vi "Redraw__LCR.vi"(8 "error in (no error)":errorcluster, 10 "BX.FP Refs":T9, 11 "State":T1={"Orientation"=0, "ActivePicture"={"image type"=0, "image depth"=0, "image"=[], "mask"=[], "colors"=[], "Rectangle"={"left"=0, "top"=0, "right"=0, "bottom"=0}}, "Pictures"={"Normal"={"image type"=0, "image depth"=0, "image"=[], "mask"=[], "colors"=[], "Rectangle"={"left"=0, "top"=0, "right"=0, "bottom"=0}}, "Hilite"={"image type"=0, "image depth"=0, "image"=[], "mask"=[], "colors"=[], "Rectangle"={"left"=0, "top"=0, "right"=0, "bottom"=0}}}, "Text"={"String"="", "Font"={"Font Name:"="", "Size"=0, "Strikeout?"=FALSE, "Italic?"=FALSE, "Underline?"=FALSE, "Outline?"=FALSE, "Shadow?"=FALSE, "Bold?"=FALSE}, "TextColor"=0}, "RunTimeSettings"={"Highlight"=FALSE, "ShowButton"=TRUE, "Behaviour"=enum."Switch when pressed", "React if disabled"=FALSE, "Nudge Button"=TRUE, "ShowButton on Hover"=FALSE, "Button Type"=enum."System"}, "Messages"=[], "Status"=0, "XControl Label"="", "Boolean Value"=FALSE} {"Status" format="%.0x"}) -> (0 "error out":errorcluster, 3 "State Out":T1={"Orientation"=0, "ActivePicture"={"image type"=0, "image depth"=0, "image"=[], "mask"=[], "colors"=[], "Rectangle"={"left"=0, "top"=0, "right"=0, "bottom"=0}}, "Pictures"={"Normal"={"image type"=0, "image depth"=0, "image"=[], "mask"=[], "colors"=[], "Rectangle"={"left"=0, "top"=0, "right"=0, "bottom"=0}}, "Hilite"={"image type"=0, "image depth"=0, "image"=[], "mask"=[], "colors"=[], "Rectangle"={"left"=0, "top"=0, "right"=0, "bottom"=0}}}, "Text"={"String"="", "Font"={"Font Name:"="", "Size"=0, "Strikeout?"=FALSE, "Italic?"=FALSE, "Underline?"=FALSE, "Outline?"=FALSE, "Shadow?"=FALSE, "Bold?"=FALSE}, "TextColor"=0}, "RunTimeSettings"={"Highlight"=FALSE, "ShowButton"=TRUE, "Behaviour"=enum."Switch when pressed", "React if disabled"=FALSE, "Nudge Button"=TRUE, "ShowButton on Hover"=FALSE, "Button Type"=enum."System"}, "Messages"=[], "Status"=0, "XControl Label"="", "Boolean Value"=FALSE} caption="State" {"Status" format="%.0x"})   [LabVIEW 2011, in "BooleanXControl__LCR.xctl"]
doc: "This VI redraws the BX"
uses:
  BooleanXControl__LCR.xctl
  Abilities/BX.State__LCR.ctl
  Controls/BX.Orientation__LCR.ctl
  <vilib>/picture/picture.llb/imagedata.ctl
  Controls/BX.RTSettings__LCR.ctl
  Controls/BX.Behaviour__LCR.ctl
  Controls/BX.ButtonType__LCR.ctl
  Controls/BX.Message__LCR.ctl
  Controls/BX.Commands__LCR.ctl
  Controls/BX.Refs__LCR.ctl
  <vilib>/Utility/miscctls.llb/LVBoundsTypeDef.ctl
  <vilib>/Utility/miscctls.llb/LVPositionTypeDef.ctl
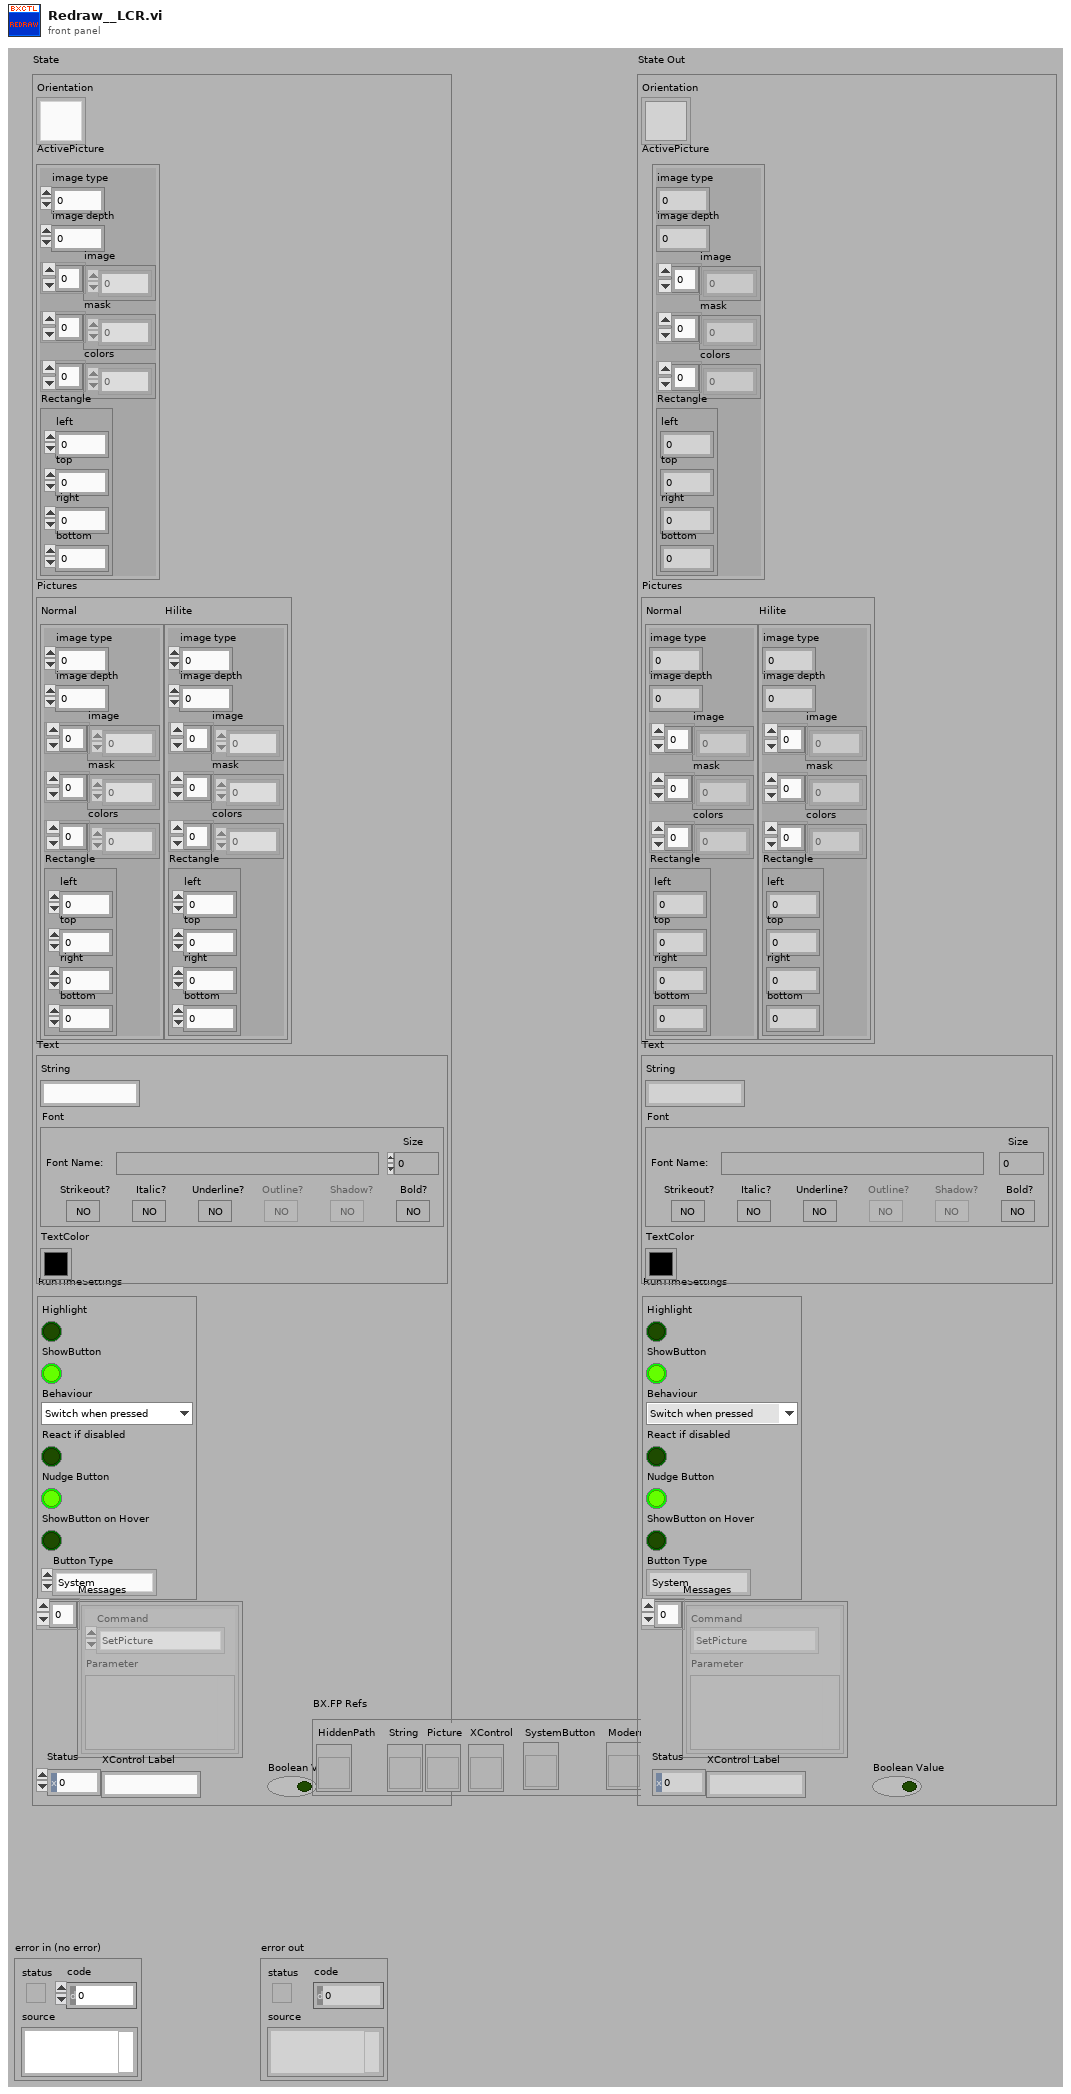
[diagram p1: front panel]
types:
  T1 = typedef "BooleanXControl__LCR.xctl/BX.State__LCR.ctl" = cluster{"Orientation":T2, "ActivePicture":T3, "Pictures":cluster{"Normal":T3, "Hilite":T3}, "Text":cluster{"String":string, "Font":cluster{"Font Name:":string, "Size":i16, "Strikeout?":bool, "Italic?":bool, "Underline?":bool, "Outline?":bool, "Shadow?":bool, "Bold?":bool}, "TextColor":u32}, "RunTimeSettings":T4, "Messages":T7[], "Status":u16, "XControl Label":string, "Boolean Value":bool}
  T2 = typedef "BooleanXControl__LCR.xctl/BX.Orientation__LCR.ctl" = u8
  T3 = typedef "imagedata.ctl" = cluster{"image type":i32, "image depth":i32, "image":u8[], "mask":u8[], "colors":u32[], "Rectangle":cluster{"left":i16, "top":i16, "right":i16, "bottom":i16}}
  T4 = typedef "BooleanXControl__LCR.xctl/BX.RTSettings__LCR.ctl" = cluster{"Highlight":bool, "ShowButton":bool, "Behaviour":T5, "React if disabled":bool, "Nudge Button":bool, "ShowButton on Hover":bool, "Button Type":T6}
  T5 = typedef "BooleanXControl__LCR.xctl/BX.Behaviour__LCR.ctl" = enum16{"Switch when pressed", "Switch when released", "Switch until released"}
  T6 = typedef "BooleanXControl__LCR.xctl/BX.ButtonType__LCR.ctl" = enum16{"System", "Modern", "Classic", "Decoration"}
  T7 = typedef "BooleanXControl__LCR.xctl/BX.Message__LCR.ctl" = cluster{"Command":T8, "Parameter":variant}
  T8 = typedef "BooleanXControl__LCR.xctl/BX.Commands__LCR.ctl" = enum16{"None", "SetPicture", "SetFont", "SetText", "SetOrientation", "Redraw", "SetTextColor", "SetRTSettings", "MultipleUpdate", "RT.Button", "RT.Hilite", "RT.Behaviour", "RT.Disabled", "ShowGUI", "RT.Nudge", "RT.Hover", "RT.ButtonType"}
  T9 = typedef "BooleanXControl__LCR.xctl/BX.Refs__LCR.ctl" = cluster{"HiddenPath":refnum<vi>, "String":refnum<vi>, "Picture":refnum<vi>, "XControl":refnum<vi>, "SystemButton":refnum<vi>, "ModernButton":refnum<vi>, "ClassicButton":refnum<vi>, "Decor Refnum":refnum<vi>}
  T10 = typedef "LVPositionTypeDef.ctl" = cluster{"Left":i32, "Top":i32}
  T11 = typedef "LVBoundsTypeDef.ctl" = cluster{"Width":u32, "Height":u32}
  T12 = cluster{"left":i16, "top":i16, "right":i16, "bottom":i16}
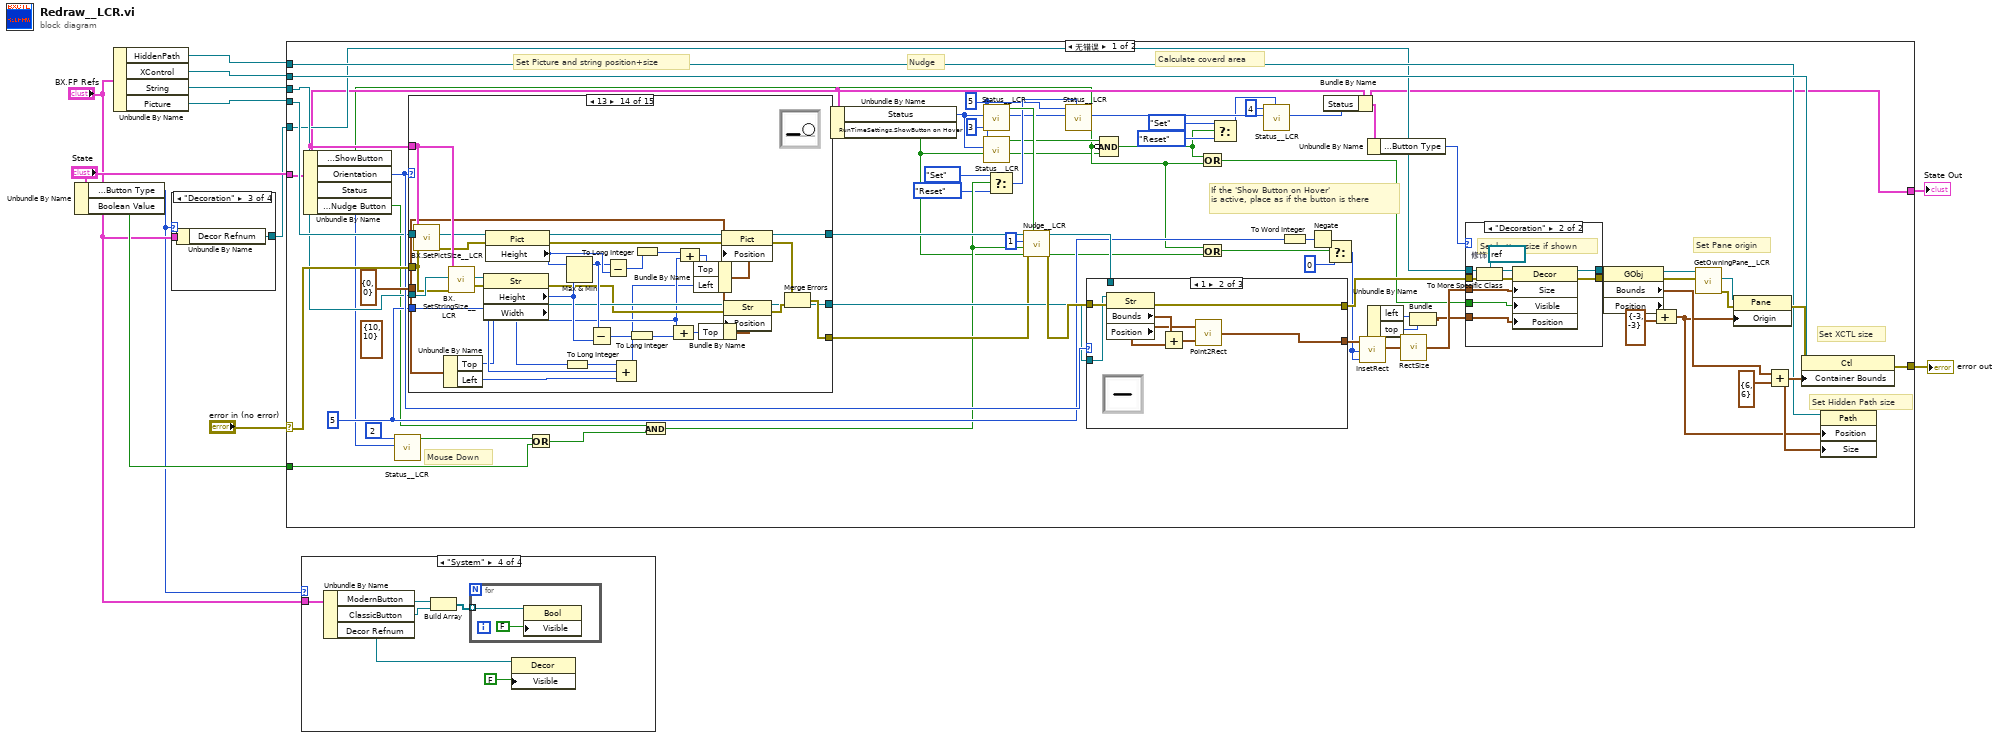
[diagram p0: block diagram]
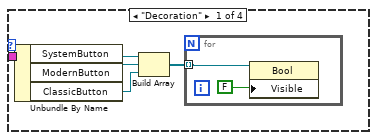
[diagram p2: hidden frame]
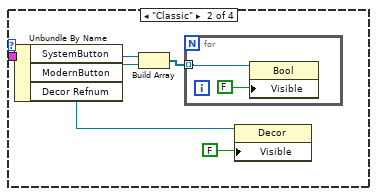
[diagram p3: hidden frame]
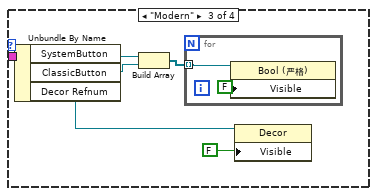
[diagram p4: hidden frame]
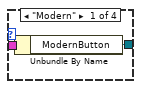
[diagram p5: hidden frame]
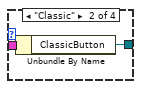
[diagram p6: hidden frame]
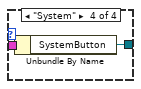
[diagram p7: hidden frame]
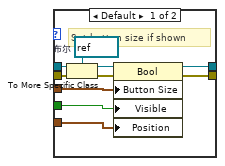
[diagram p8: hidden frame]
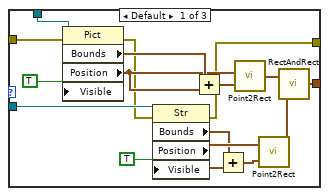
[diagram p9: hidden frame]
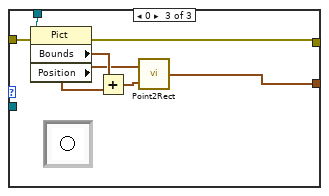
[diagram p10: hidden frame]
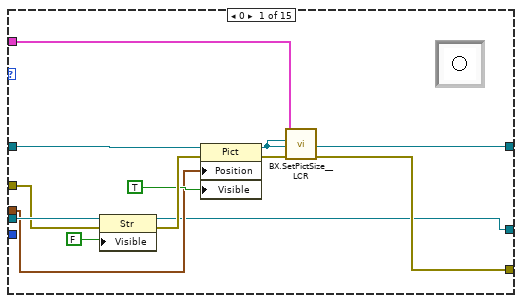
[diagram p11: hidden frame]
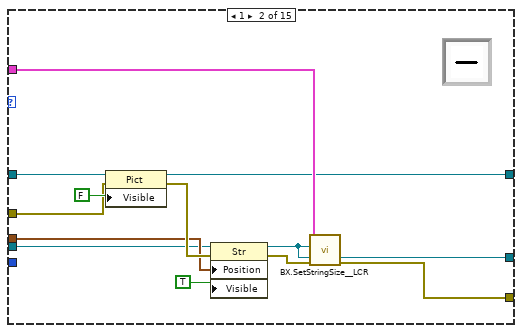
[diagram p12: hidden frame]
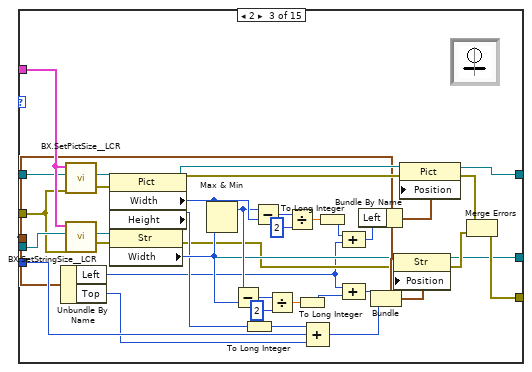
[diagram p13: hidden frame]
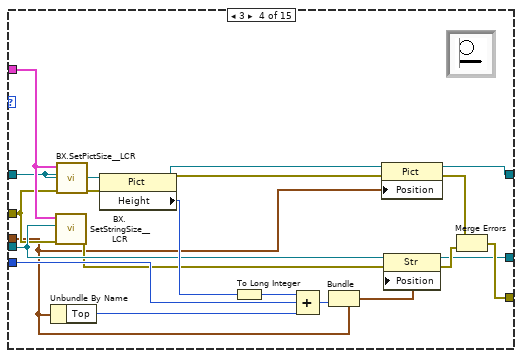
[diagram p14: hidden frame]
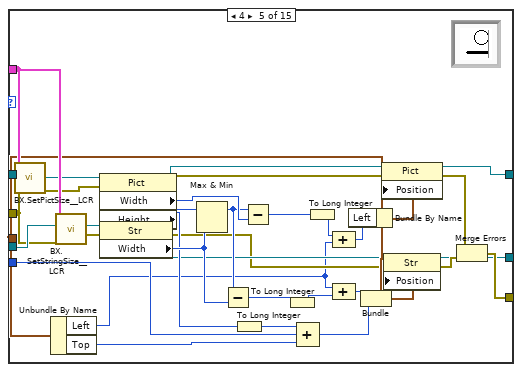
[diagram p15: hidden frame]
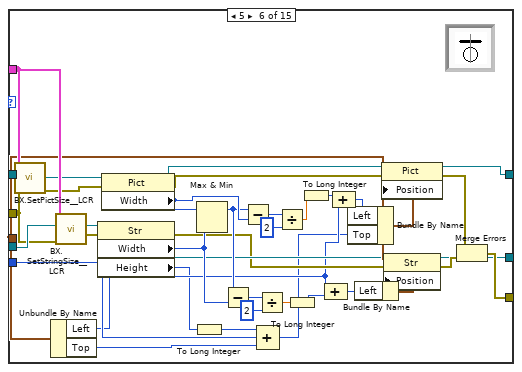
[diagram p16: hidden frame]
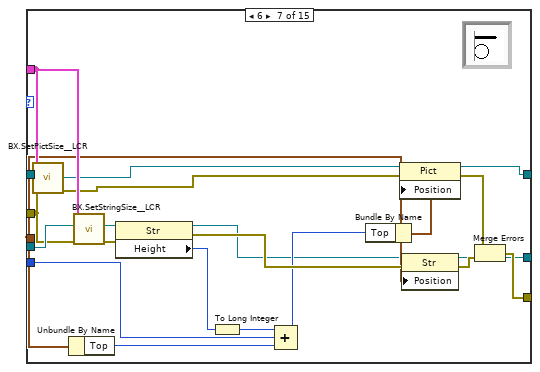
[diagram p17: hidden frame]
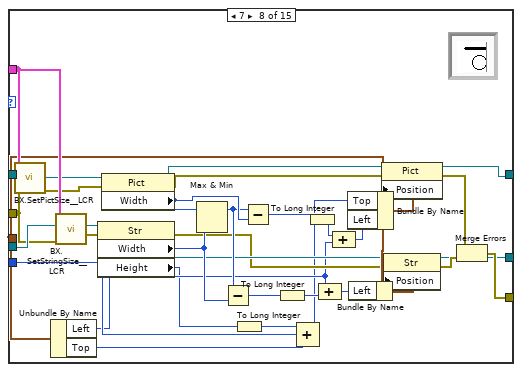
[diagram p18: hidden frame]
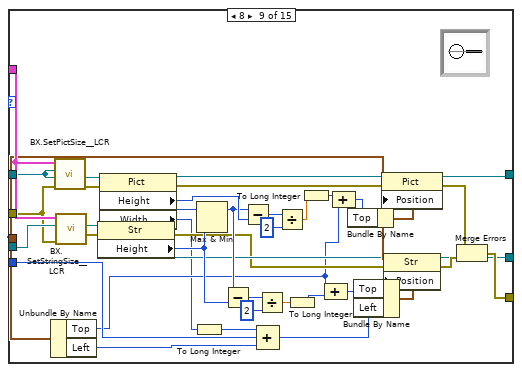
[diagram p19: hidden frame]
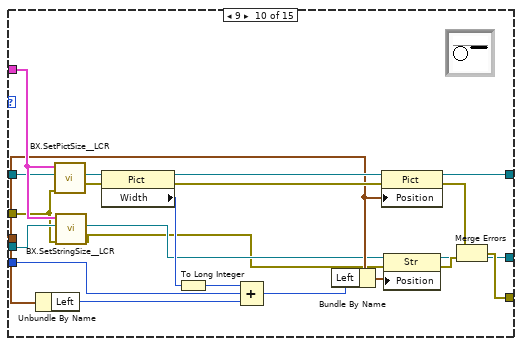
[diagram p20: hidden frame]
diagram:
  n1 = Unbundle By Name("State") -> ("RunTimeSettings.Button Type"=w1:T6, "Boolean Value"=w3:bool)
  n2 = Unbundle By Name("BX.FP Refs") -> ("HiddenPath"=w7:refnum<vi>, "XControl"=w8:refnum<vi>, "String"=w9:refnum<vi>, "Picture"=w10:refnum<vi>)
  n3 = case shown="\"Decoration\"" w1 {
    tunnel: "BX.FP Refs" -> [w14 w16 w18 w20]
    tunnel: [w13 w15 w17 w19] -> w4
    frame "Modern" {
      n4 = Unbundle By Name(w14) -> ("ModernButton"=w13:refnum<vi>)
    }
    frame "Classic" {
      n5 = Unbundle By Name(w16) -> ("ClassicButton"=w15:refnum<vi>)
    }
    frame "Decoration" {
      n6 = Unbundle By Name(w18) -> ("Decor Refnum"=w17:refnum<vi>)
    }
    frame "System" {
      n7 = Unbundle By Name(w20) -> ("SystemButton"=w19:refnum<vi>)
    }
  }
  n8 = case shown="无错误" "error in (no error)" {
    selector: "error in (no error)" -> [w74 w529]
    tunnel: [w77 w529] -> w11
    tunnel: "State" -> [w49 w528]
    tunnel: w10 -> [w62 _]
    tunnel: w4 -> [w51 _]
    tunnel: w9 -> [w61 _]
    tunnel: w8 -> [w66 _]
    tunnel: w7 -> [w65 _]
    tunnel: [w23 w528] -> w6
    tunnel: w3 -> [w21 _]
    frame No Error {
      (unwired) T10 {"Left"=10, "Top"=10} ("Position")
      w31 = u16 5 ("Bit")
      w56 = 5
      # "If the 'Show Button on Hover' \nis active, place as if the button is there"
      # "Mouse Down"
      # "Nudge"
      # "Set XCTL size"
      # "Set Hidden Path size"
      # "Set Pane origin"
      # "Calculate coverd area"
      # "Set Picture and string position+size"
      n9 = Unbundle By Name(w49) -> ("RunTimeSettings.ShowButton"=w27:bool, "Orientation"=w64:T2, "Status"=w53:u16, "RunTimeSettings.Nudge Button"=w52:bool)
      n10 = call "Status__LCR.vi"("Status In"=w53, "Bit"=u16 2 ("y")) -> ("Bit Value Out"=w24:bool)  [unwired: 8 in, 1 out]
      n11 = case shown="13" w64 {
        tunnel: w61 -> [w152 w155 w200 w208 w253 w290 w310 w343 w380 w386 w433 w470 w479 w523 w525]
        tunnel: w74 -> [w150 w163 w167 w205 w224 w257 w294 w314 w347 w384 w404 w437 w474 w494 w527]
        tunnel: T10 {"Left"=0, "Top"=0} ("Position") -> [w143 w161 w182 w204 w241 w273 w296 w332 w363 w387 w422 w453 w481 w512 _]
        tunnel: w62 -> [w148 w156 w198 w220 w251 w288 w299 w341 w378 w400 w431 w468 w480 w521 w526]
        tunnel: w49 -> [w146 w159 w201 w221 w254 w291 w311 w344 w381 w401 w434 w471 w491 w524 _]
        tunnel: [w144 w157 w175 w211 w234 w267 w304 w326 w357 w392 w416 w447 w487 w506 w527] -> w55
        tunnel: w56 -> [_ _ w184 w216 w243 w275 w308 w334 w365 w396 w424 w455 w490 w514 _]
        tunnel: [w142 w154 w166 w203 w223 w256 w293 w313 w346 w383 w403 w436 w473 w493 w526] -> w58
        tunnel: [w141 w153 w165 w202 w222 w255 w292 w312 w345 w382 w402 w435 w472 w492 w525] -> w60
        frame 0 {
          n12 = property class="Str"(reference=w152, error in=w150, "Visible"=FALSE) -> (reference out=w141:refnum<vi>, error out=w149:errorcluster)
          n13 = property class="Pict"(reference=w148, error in=w149, "Position"=w143, "Visible"=TRUE) -> (reference out=w142:refnum<vi>, error out=w145:errorcluster)
          n14 = call "BX.SetPictSize__LCR.vi"("error in (no error)"=w145, "Picture Control"=w142, "State"=w146) -> ("error out"=w144:errorcluster)  [unwired: 8 in]
        }
        frame 1 {
          n15 = property class="Pict"(reference=w156, error in=w163, "Visible"=FALSE) -> (reference out=w154:refnum<vi>, error out=w162:errorcluster)
          n16 = property class="Str"(reference=w155, error in=w162, "Position"=w161, "Visible"=TRUE) -> (reference out=w153:refnum<vi>, error out=w158:errorcluster)
          n17 = call "BX.SetStringSize__LCR.vi"("error in (no error)"=w158, "String Control"=w153, "State"=w159) -> ("error out"=w157:errorcluster)  [unwired: 8 in]
        }
        frame 2 {
          n18 = Unbundle By Name(w182) -> ("Left"=w168:i32, "Top"=w183:i32)
          n19 = call "BX.SetPictSize__LCR.vi"("error in (no error)"=w167, "Picture Control"=w198, "State"=w201) -> ("error out"=w197:errorcluster)  [unwired: 8 in]
          n20 = call "BX.SetStringSize__LCR.vi"("error in (no error)"=w167, "String Control"=w200, "State"=w201) -> ("error out"=w199:errorcluster)  [unwired: 8 in]
          n21 = property class="Pict"(reference=w198, error in=w197) -> (reference out=w187:refnum<vi>, error out=w186:errorcluster, "Width"=w196:u32, "Height"=w185:u32)
          n22 = property class="Str"(reference=w200, error in=w199) -> (reference out=w178:refnum<vi>, error out=w177:errorcluster, "Width"=w190:u32)
          n23 = Max & Min(x=w196, y=w190) -> (max(x,y)=w191:u32)  [unwired: 1 out]
          n24 = Subtract(x=w191, y=w190) -> (x-y=w192:u32)
          n25 = To Long Integer(number=w185) -> (32bit integer=w180:i32)
          n26 = Subtract(x=w191, y=w196) -> (x-y=w195:u32)
          n27 = Divide(x=w192, y=u32 2) -> (x/y=w188:dbl)
          n28 = Divide(x=w195, y=u32 2) -> (x/y=w189:dbl)
          n29 = To Long Integer(number=w188) -> (32bit integer=w170:i32)
          n30 = Compound Arithmetic op=ADD(w180, w184, w183) -> (w181:i32)
          n31 = To Long Integer(number=w189) -> (32bit integer=w172:i32)
          n32 = Compound Arithmetic op=ADD(w172, w168) -> (w171:i32)
          n33 = Compound Arithmetic op=ADD(w168, w170) -> (w169:i32)
          n34 = Bundle By Name(cluster=w182, "Left"=w171) -> (w179:T10)
          n35 = Bundle(cluster=w182, "Left"=w169, "Top"=w181) -> (w176:T10)
          n36 = property class="Str"(reference=w178, error in=w177, "Position"=w176) -> (reference out=w165:refnum<vi>, error out=w173:errorcluster)
          n37 = property class="Pict"(reference=w187, error in=w186, "Position"=w179) -> (reference out=w166:refnum<vi>, error out=w174:errorcluster)
          n38 = Merge Errors(w174, w173) -> (w175:errorcluster)
        }
        frame 3 {
          n39 = Unbundle By Name(w204) -> ("Top"=w215:i32)
          n40 = call "BX.SetStringSize__LCR.vi"("error in (no error)"=w205, "String Control"=w208, "State"=w221) -> ("error out"=w207:errorcluster)  [unwired: 8 in]
          n41 = call "BX.SetPictSize__LCR.vi"("error in (no error)"=w205, "Picture Control"=w220, "State"=w221) -> ("error out"=w206:errorcluster)  [unwired: 8 in]
          n42 = property class="Pict"(reference=w220, error in=w206) -> (reference out=w219:refnum<vi>, error out=w218:errorcluster, "Height"=w217:u32)
          n43 = To Long Integer(number=w217) -> (32bit integer=w213:i32)
          n44 = Compound Arithmetic op=ADD(w213, w216, w215) -> (w214:i32)
          n45 = Bundle(cluster=w204, "Top"=w214) -> (w212:T10)  [unwired: 1 in]
          n46 = property class="Pict"(reference=w219, error in=w218, "Position"=w204) -> (reference out=w203:refnum<vi>, error out=w210:errorcluster)
          n47 = property class="Str"(reference=w208, error in=w207, "Position"=w212) -> (reference out=w202:refnum<vi>, error out=w209:errorcluster)
          n48 = Merge Errors(w210, w209) -> (w211:errorcluster)
        }
        frame 4 {
          n49 = call "BX.SetPictSize__LCR.vi"("error in (no error)"=w224, "Picture Control"=w251, "State"=w254) -> ("error out"=w250:errorcluster)  [unwired: 8 in]
          n50 = Unbundle By Name(w241) -> ("Left"=w227:i32, "Top"=w242:i32)
          n51 = call "BX.SetStringSize__LCR.vi"("error in (no error)"=w224, "String Control"=w253, "State"=w254) -> ("error out"=w252:errorcluster)  [unwired: 8 in]
          n52 = property class="Pict"(reference=w251, error in=w250) -> (reference out=w246:refnum<vi>, error out=w245:errorcluster, "Width"=w249:u32, "Height"=w244:u32)
          n53 = property class="Str"(reference=w253, error in=w252) -> (reference out=w237:refnum<vi>, error out=w236:errorcluster, "Width"=w247:u32)
          n54 = Max & Min(x=w249, y=w247) -> (max(x,y)=w248:u32)  [unwired: 1 out]
          n55 = Subtract(x=w248, y=w247) -> (x-y=w225:u32)
          n56 = To Long Integer(number=w244) -> (32bit integer=w239:i32)
          n57 = Subtract(x=w248, y=w249) -> (x-y=w226:u32)
          n58 = To Long Integer(number=w225) -> (32bit integer=w229:i32)
          n59 = Compound Arithmetic op=ADD(w239, w243, w242) -> (w240:i32)
          n60 = To Long Integer(number=w226) -> (32bit integer=w231:i32)
          n61 = Compound Arithmetic op=ADD(w231, w227) -> (w230:i32)
          n62 = Compound Arithmetic op=ADD(w227, w229) -> (w228:i32)
          n63 = Bundle By Name(cluster=w241, "Left"=w230) -> (w238:T10)
          n64 = Bundle(cluster=w241, "Left"=w228, "Top"=w240) -> (w235:T10)
          n65 = property class="Pict"(reference=w246, error in=w245, "Position"=w238) -> (reference out=w223:refnum<vi>, error out=w233:errorcluster)
          n66 = property class="Str"(reference=w237, error in=w236, "Position"=w235) -> (reference out=w222:refnum<vi>, error out=w232:errorcluster)
          n67 = Merge Errors(w233, w232) -> (w234:errorcluster)
        }
        frame 5 {
          n68 = call "BX.SetPictSize__LCR.vi"("error in (no error)"=w257, "Picture Control"=w288, "State"=w291) -> ("error out"=w287:errorcluster)  [unwired: 8 in]
          n69 = Unbundle By Name(w273) -> ("Left"=w260:i32, "Top"=w274:i32)
          n70 = call "BX.SetStringSize__LCR.vi"("error in (no error)"=w257, "String Control"=w290, "State"=w291) -> ("error out"=w289:errorcluster)  [unwired: 8 in]
          n71 = property class="Str"(reference=w290, error in=w289) -> (reference out=w270:refnum<vi>, error out=w269:errorcluster, "Width"=w280:u32, "Height"=w259:u32)
          n72 = property class="Pict"(reference=w288, error in=w287) -> (reference out=w277:refnum<vi>, error out=w276:errorcluster, "Width"=w286:u32)
          n73 = To Long Integer(number=w259) -> (32bit integer=w272:i32)
          n74 = Max & Min(x=w286, y=w280) -> (max(x,y)=w281:u32)  [unwired: 1 out]
          n75 = Subtract(x=w281, y=w280) -> (x-y=w282:u32)
          n76 = Subtract(x=w281, y=w286) -> (x-y=w285:u32)
          n77 = Divide(x=w282, y=u32 2) -> (x/y=w278:dbl)
          n78 = Compound Arithmetic op=ADD(w272, w275, w274) -> (w258:i32)
          n79 = Divide(x=w285, y=u32 2) -> (x/y=w279:dbl)
          n80 = To Long Integer(number=w278) -> (32bit integer=w262:i32)
          n81 = To Long Integer(number=w279) -> (32bit integer=w264:i32)
          n82 = Compound Arithmetic op=ADD(w260, w262) -> (w261:i32)
          n83 = Compound Arithmetic op=ADD(w264, w260) -> (w263:i32)
          n84 = Bundle By Name(cluster=w273, "Left"=w263, "Top"=w258) -> (w271:T10)
          n85 = Bundle By Name(cluster=w273, "Left"=w261) -> (w268:T10)
          n86 = property class="Pict"(reference=w277, error in=w276, "Position"=w271) -> (reference out=w256:refnum<vi>, error out=w266:errorcluster)
          n87 = property class="Str"(reference=w270, error in=w269, "Position"=w268) -> (reference out=w255:refnum<vi>, error out=w265:errorcluster)
          n88 = Merge Errors(w266, w265) -> (w267:errorcluster)
        }
        frame 6 {
          n89 = call "BX.SetPictSize__LCR.vi"("error in (no error)"=w294, "Picture Control"=w299, "State"=w311) -> ("error out"=w298:errorcluster)  [unwired: 8 in]
          n90 = Unbundle By Name(w296) -> ("Top"=w307:i32)
          n91 = call "BX.SetStringSize__LCR.vi"("error in (no error)"=w294, "String Control"=w310, "State"=w311) -> ("error out"=w309:errorcluster)  [unwired: 8 in]
          n92 = property class="Str"(reference=w310, error in=w309) -> (reference out=w295:refnum<vi>, error out=w300:errorcluster, "Height"=w301:u32)
          n93 = To Long Integer(number=w301) -> (32bit integer=w306:i32)
          n94 = Compound Arithmetic op=ADD(w306, w308, w307) -> (w297:i32)
          n95 = Bundle By Name(cluster=w296, "Top"=w297) -> (w305:T10)
          n96 = property class="Pict"(reference=w299, error in=w298, "Position"=w305) -> (reference out=w293:refnum<vi>, error out=w303:errorcluster)
          n97 = property class="Str"(reference=w295, error in=w300, "Position"=w296) -> (reference out=w292:refnum<vi>, error out=w302:errorcluster)
          n98 = Merge Errors(w303, w302) -> (w304:errorcluster)
        }
        frame 7 {
          n99 = call "BX.SetPictSize__LCR.vi"("error in (no error)"=w314, "Picture Control"=w341, "State"=w344) -> ("error out"=w340:errorcluster)  [unwired: 8 in]
          n100 = Unbundle By Name(w332) -> ("Left"=w319:i32, "Top"=w333:i32)
          n101 = call "BX.SetStringSize__LCR.vi"("error in (no error)"=w314, "String Control"=w343, "State"=w344) -> ("error out"=w342:errorcluster)  [unwired: 8 in]
          n102 = property class="Str"(reference=w343, error in=w342) -> (reference out=w329:refnum<vi>, error out=w328:errorcluster, "Width"=w337:u32, "Height"=w315:u32)
          n103 = property class="Pict"(reference=w341, error in=w340) -> (reference out=w336:refnum<vi>, error out=w335:errorcluster, "Width"=w339:u32)
          n104 = Max & Min(x=w339, y=w337) -> (max(x,y)=w338:u32)  [unwired: 1 out]
          n105 = Subtract(x=w338, y=w337) -> (x-y=w317:u32)
          n106 = To Long Integer(number=w315) -> (32bit integer=w331:i32)
          n107 = Subtract(x=w338, y=w339) -> (x-y=w318:u32)
          n108 = To Long Integer(number=w317) -> (32bit integer=w321:i32)
          n109 = Compound Arithmetic op=ADD(w331, w334, w333) -> (w316:i32)
          n110 = To Long Integer(number=w318) -> (32bit integer=w323:i32)
          n111 = Compound Arithmetic op=ADD(w319, w321) -> (w320:i32)
          n112 = Compound Arithmetic op=ADD(w323, w319) -> (w322:i32)
          n113 = Bundle By Name(cluster=w332, "Top"=w316, "Left"=w322) -> (w330:T10)
          n114 = Bundle By Name(cluster=w332, "Left"=w320) -> (w327:T10)
          n115 = property class="Pict"(reference=w336, error in=w335, "Position"=w330) -> (reference out=w313:refnum<vi>, error out=w325:errorcluster)
          n116 = property class="Str"(reference=w329, error in=w328, "Position"=w327) -> (reference out=w312:refnum<vi>, error out=w324:errorcluster)
          n117 = Merge Errors(w325, w324) -> (w326:errorcluster)
        }
        frame 8 {
          n118 = Unbundle By Name(w363) -> ("Top"=w350:i32, "Left"=w364:i32)
          n119 = call "BX.SetPictSize__LCR.vi"("error in (no error)"=w347, "Picture Control"=w378, "State"=w381) -> ("error out"=w377:errorcluster)  [unwired: 8 in]
          n120 = call "BX.SetStringSize__LCR.vi"("error in (no error)"=w347, "String Control"=w380, "State"=w381) -> ("error out"=w379:errorcluster)  [unwired: 8 in]
          n121 = property class="Str"(reference=w380, error in=w379) -> (reference out=w360:refnum<vi>, error out=w359:errorcluster, "Height"=w370:u32)
          n122 = property class="Pict"(reference=w378, error in=w377) -> (reference out=w367:refnum<vi>, error out=w366:errorcluster, "Height"=w376:u32, "Width"=w349:u32)
          n123 = To Long Integer(number=w349) -> (32bit integer=w362:i32)
          n124 = Max & Min(x=w376, y=w370) -> (max(x,y)=w371:u32)  [unwired: 1 out]
          n125 = Subtract(x=w371, y=w370) -> (x-y=w372:u32)
          n126 = Subtract(x=w371, y=w376) -> (x-y=w375:u32)
          n127 = Divide(x=w372, y=u32 2) -> (x/y=w368:dbl)
          n128 = Compound Arithmetic op=ADD(w362, w365, w364) -> (w348:i32)
          n129 = Divide(x=w375, y=u32 2) -> (x/y=w369:dbl)
          n130 = To Long Integer(number=w368) -> (32bit integer=w352:i32)
          n131 = To Long Integer(number=w369) -> (32bit integer=w354:i32)
          n132 = Compound Arithmetic op=ADD(w350, w352) -> (w351:i32)
          n133 = Compound Arithmetic op=ADD(w354, w350) -> (w353:i32)
          n134 = Bundle By Name(cluster=w363, "Top"=w353) -> (w361:T10)
          n135 = Bundle By Name(cluster=w363, "Top"=w351, "Left"=w348) -> (w358:T10)
          n136 = property class="Pict"(reference=w367, error in=w366, "Position"=w361) -> (reference out=w346:refnum<vi>, error out=w356:errorcluster)
          n137 = property class="Str"(reference=w360, error in=w359, "Position"=w358) -> (reference out=w345:refnum<vi>, error out=w355:errorcluster)
          n138 = Merge Errors(w356, w355) -> (w357:errorcluster)
        }
        frame 9 {
          n139 = Unbundle By Name(w387) -> ("Left"=w395:i32)
          n140 = call "BX.SetPictSize__LCR.vi"("error in (no error)"=w384, "Picture Control"=w400, "State"=w401) -> ("error out"=w399:errorcluster)  [unwired: 8 in]
          n141 = call "BX.SetStringSize__LCR.vi"("error in (no error)"=w384, "String Control"=w386, "State"=w401) -> ("error out"=w385:errorcluster)  [unwired: 8 in]
          n142 = property class="Pict"(reference=w400, error in=w399) -> (reference out=w398:refnum<vi>, error out=w397:errorcluster, "Width"=w389:u32)
          n143 = To Long Integer(number=w389) -> (32bit integer=w394:i32)
          n144 = Compound Arithmetic op=ADD(w394, w396, w395) -> (w388:i32)
          n145 = Bundle By Name(cluster=w387, "Left"=w388) -> (w393:T10)
          n146 = property class="Pict"(reference=w398, error in=w397, "Position"=w387) -> (reference out=w383:refnum<vi>, error out=w391:errorcluster)
          n147 = property class="Str"(reference=w386, error in=w385, "Position"=w393) -> (reference out=w382:refnum<vi>, error out=w390:errorcluster)
          n148 = Merge Errors(w391, w390) -> (w392:errorcluster)
        }
        frame 10 {
          n149 = call "BX.SetPictSize__LCR.vi"("error in (no error)"=w404, "Picture Control"=w431, "State"=w434) -> ("error out"=w430:errorcluster)  [unwired: 8 in]
          n150 = Unbundle By Name(w422) -> ("Top"=w409:i32, "Left"=w423:i32)
          n151 = call "BX.SetStringSize__LCR.vi"("error in (no error)"=w404, "String Control"=w433, "State"=w434) -> ("error out"=w432:errorcluster)  [unwired: 8 in]
          n152 = property class="Str"(reference=w433, error in=w432) -> (reference out=w419:refnum<vi>, error out=w418:errorcluster, "Height"=w427:u32)
          n153 = property class="Pict"(reference=w431, error in=w430) -> (reference out=w426:refnum<vi>, error out=w425:errorcluster, "Height"=w429:u32, "Width"=w408:u32)
          n154 = To Long Integer(number=w408) -> (32bit integer=w421:i32)
          n155 = Max & Min(x=w429, y=w427) -> (max(x,y)=w428:u32)  [unwired: 1 out]
          n156 = Subtract(x=w428, y=w427) -> (x-y=w405:u32)
          n157 = Subtract(x=w428, y=w429) -> (x-y=w406:u32)
          n158 = Compound Arithmetic op=ADD(w421, w424, w423) -> (w407:i32)
          n159 = To Long Integer(number=w405) -> (32bit integer=w411:i32)
          n160 = To Long Integer(number=w406) -> (32bit integer=w413:i32)
          n161 = Compound Arithmetic op=ADD(w413, w409) -> (w412:i32)
          n162 = Compound Arithmetic op=ADD(w409, w411) -> (w410:i32)
          n163 = Bundle By Name(cluster=w422, "Top"=w412) -> (w420:T10)
          n164 = Bundle By Name(cluster=w422, "Top"=w410, "Left"=w407) -> (w417:T10)
          n165 = property class="Pict"(reference=w426, error in=w425, "Position"=w420) -> (reference out=w403:refnum<vi>, error out=w415:errorcluster)
          n166 = property class="Str"(reference=w419, error in=w418, "Position"=w417) -> (reference out=w402:refnum<vi>, error out=w414:errorcluster)
          n167 = Merge Errors(w415, w414) -> (w416:errorcluster)
        }
        frame 11 {
          n168 = call "BX.SetPictSize__LCR.vi"("error in (no error)"=w437, "Picture Control"=w468, "State"=w471) -> ("error out"=w467:errorcluster)  [unwired: 8 in]
          n169 = Unbundle By Name(w453) -> ("Top"=w440:i32, "Left"=w454:i32)
          n170 = call "BX.SetStringSize__LCR.vi"("error in (no error)"=w437, "String Control"=w470, "State"=w471) -> ("error out"=w469:errorcluster)  [unwired: 8 in]
          n171 = property class="Str"(reference=w470, error in=w469) -> (reference out=w450:refnum<vi>, error out=w449:errorcluster, "Height"=w460:u32, "Width"=w439:u32)
          n172 = property class="Pict"(reference=w468, error in=w467) -> (reference out=w457:refnum<vi>, error out=w456:errorcluster, "Height"=w466:u32)
          n173 = To Long Integer(number=w439) -> (32bit integer=w452:i32)
          n174 = Max & Min(x=w466, y=w460) -> (max(x,y)=w461:u32)  [unwired: 1 out]
          n175 = Subtract(x=w461, y=w460) -> (x-y=w462:u32)
          n176 = Subtract(x=w461, y=w466) -> (x-y=w465:u32)
          n177 = Divide(x=w462, y=u32 2) -> (x/y=w458:dbl)
          n178 = Compound Arithmetic op=ADD(w452, w455, w454) -> (w438:i32)
          n179 = Divide(x=w465, y=u32 2) -> (x/y=w459:dbl)
          n180 = To Long Integer(number=w458) -> (32bit integer=w442:i32)
          n181 = To Long Integer(number=w459) -> (32bit integer=w444:i32)
          n182 = Compound Arithmetic op=ADD(w440, w442) -> (w441:i32)
          n183 = Compound Arithmetic op=ADD(w444, w440) -> (w443:i32)
          n184 = Bundle By Name(cluster=w453, "Top"=w443, "Left"=w438) -> (w451:T10)
          n185 = Bundle By Name(cluster=w453, "Top"=w441) -> (w448:T10)
          n186 = property class="Pict"(reference=w457, error in=w456, "Position"=w451) -> (reference out=w436:refnum<vi>, error out=w446:errorcluster)
          n187 = property class="Str"(reference=w450, error in=w449, "Position"=w448) -> (reference out=w435:refnum<vi>, error out=w445:errorcluster)
          n188 = Merge Errors(w446, w445) -> (w447:errorcluster)
        }
        frame 12 {
          n189 = call "BX.SetPictSize__LCR.vi"("error in (no error)"=w474, "Picture Control"=w480, "State"=w491) -> ("error out"=w477:errorcluster)  [unwired: 8 in]
          n190 = Unbundle By Name(w481) -> ("Left"=w489:i32)
          n191 = call "BX.SetStringSize__LCR.vi"("error in (no error)"=w474, "String Control"=w479, "State"=w491) -> ("error out"=w476:errorcluster)  [unwired: 8 in]
          n192 = property class="Str"(reference=w479, error in=w476) -> (reference out=w478:refnum<vi>, error out=w475:errorcluster, "Width"=w484:u32)
          n193 = To Long Integer(number=w484) -> (32bit integer=w488:i32)
          n194 = Compound Arithmetic op=ADD(w488, w490, w489) -> (w483:i32)
          n195 = Bundle By Name(cluster=w481, "Left"=w483) -> (w482:T10)
          n196 = property class="Pict"(reference=w480, error in=w477, "Position"=w482) -> (reference out=w473:refnum<vi>, error out=w486:errorcluster)
          n197 = property class="Str"(reference=w478, error in=w475, "Position"=w481) -> (reference out=w472:refnum<vi>, error out=w485:errorcluster)
          n198 = Merge Errors(w486, w485) -> (w487:errorcluster)
        }
        frame 13 {
          n199 = call "BX.SetPictSize__LCR.vi"("error in (no error)"=w494, "Picture Control"=w521, "State"=w524) -> ("error out"=w520:errorcluster)  [unwired: 8 in]
          n200 = Unbundle By Name(w512) -> ("Top"=w499:i32, "Left"=w513:i32)
          n201 = call "BX.SetStringSize__LCR.vi"("error in (no error)"=w494, "String Control"=w523, "State"=w524) -> ("error out"=w522:errorcluster)  [unwired: 8 in]
          n202 = property class="Str"(reference=w523, error in=w522) -> (reference out=w509:refnum<vi>, error out=w508:errorcluster, "Height"=w517:u32, "Width"=w496:u32)
          n203 = property class="Pict"(reference=w521, error in=w520) -> (reference out=w516:refnum<vi>, error out=w515:errorcluster, "Height"=w519:u32)
          n204 = To Long Integer(number=w496) -> (32bit integer=w511:i32)
          n205 = Max & Min(x=w519, y=w517) -> (max(x,y)=w518:u32)  [unwired: 1 out]
          n206 = Subtract(x=w518, y=w517) -> (x-y=w497:u32)
          n207 = Subtract(x=w518, y=w519) -> (x-y=w498:u32)
          n208 = Compound Arithmetic op=ADD(w511, w514, w513) -> (w495:i32)
          n209 = To Long Integer(number=w497) -> (32bit integer=w501:i32)
          n210 = To Long Integer(number=w498) -> (32bit integer=w503:i32)
          n211 = Compound Arithmetic op=ADD(w499, w501) -> (w500:i32)
          n212 = Compound Arithmetic op=ADD(w503, w499) -> (w502:i32)
          n213 = Bundle By Name(cluster=w512, "Top"=w502, "Left"=w495) -> (w510:T10)
          n214 = Bundle By Name(cluster=w512, "Top"=w500) -> (w507:T10)
          n215 = property class="Pict"(reference=w516, error in=w515, "Position"=w510) -> (reference out=w493:refnum<vi>, error out=w505:errorcluster)
          n216 = property class="Str"(reference=w509, error in=w508, "Position"=w507) -> (reference out=w492:refnum<vi>, error out=w504:errorcluster)
          n217 = Merge Errors(w505, w504) -> (w506:errorcluster)
        }
        frame Default {
        }
      }
      n218 = Or(x=w24, y=w21) -> (x .or. y?=w50:bool)
      n219 = And(x=w52, y=w50) -> (x .and. y?=w47:bool)
      n220 = Unbundle By Name(w49) -> ("Status"=w42:u16, "RunTimeSettings.ShowButton on Hover"=w26:bool)
      n221 = call "Status__LCR.vi"("Status In"=w42, "Bit"=w31) -> ("Status Out"=w43:u16, "Bit Value Out"=w48:bool)  [unwired: 8 in]
      n222 = call "Status__LCR.vi"("Status In"=w42, "Bit"=u16 3) -> ("Bit Value Out"=w40:bool)  [unwired: 8 in, 1 out]
      n223 = Select(t=enum16{"Get", "Set", "Reset"}."Set" ("Action (Get)"), s=w47, f=enum16{"Get", "Set", "Reset"}."Reset" ("Action (Get)")) -> (s? t:f=w44:enum16{"Get", "Set", "Reset"})
      n224 = call "Nudge__LCR.vi"("Nudging?"=w48, "error in (no error)"=w55, "Nudge?"=w47, "NudgeValue"=1, "Pict In"=w58) -> ("error out"=w63:errorcluster, "PictOut"=w57:refnum<vi>)  [unwired: 5 in]
      n225 = call "Status__LCR.vi"("Action (Get)"=w44, "Status In"=w43, "Bit"=w31) -> ("Status Out"=w37:u16)  [unwired: 7 in, 1 out]
      n226 = case shown="1" w64 {
        tunnel: w63 -> [w126 w133 w140]
        tunnel: w57 -> [w125 _ w139]
        tunnel: w60 -> [w119 w127 _]
        tunnel: [w115 w129 w135] -> w73
        tunnel: [w114 w128 w134] -> w88
        frame Default {
          n227 = property class="Pict"(reference=w125, error in=w126, "Visible"=TRUE) -> (error out=w118:errorcluster, "Bounds"=w124:T11, "Position"=w123:T10)  [unwired: 1 out]
          n228 = property class="Str"(reference=w119, error in=w118, "Visible"=TRUE) -> (error out=w114:errorcluster, "Bounds"=w111:T11, "Position"=w120:T10)  [unwired: 1 out]
          n229 = Add(x=w124, y=w123) -> (x+y=w122:T11)
          n230 = Add(x=w111, y=w120) -> (x+y=w121:T11)
          n231 = call <vilib>:"Point2Rect.vi"("point b"=w122, "point a"=w123) -> ("rect"=w117:T12)
          n232 = call <vilib>:"Point2Rect.vi"("point b"=w121, "point a"=w120) -> ("rect"=w116:T12)
          n233 = call <vilib>:"RectAndRect.vi"("rect b"=w116, "rect a"=w117) -> ("union rect"=w115:T12)
        }
        frame 1 {
          n234 = property class="Str"(reference=w127, error in=w133) -> (error out=w128:errorcluster, "Bounds"=w132:T11, "Position"=w131:T10)  [unwired: 1 out]
          n235 = Add(x=w132, y=w131) -> (x+y=w130:T11)
          n236 = call <vilib>:"Point2Rect.vi"("point b"=w130, "point a"=w131) -> ("rect"=w129:T12)
        }
        frame 0 {
          n237 = property class="Pict"(reference=w139, error in=w140) -> (error out=w134:errorcluster, "Bounds"=w138:T11, "Position"=w137:T10)  [unwired: 1 out]
          n238 = Add(x=w138, y=w137) -> (x+y=w136:T11)
          n239 = call <vilib>:"Point2Rect.vi"("point b"=w136, "point a"=w137) -> ("rect"=w135:T12)
        }
      }
      n240 = Compound Arithmetic op=AND(w40, invert w27, w26) -> (w33:bool)
      n241 = Or(x=w33, y=w27) -> (x .or. y?=w32:bool)
      n242 = Or(x=w27, y=w26) -> (x .or. y?=w25:bool)
      n243 = Select(t=enum16{"Get", "Set", "Reset"}."Set" ("Action (Get)"), s=w33, f=enum16{"Get", "Set", "Reset"}."Reset" ("Action (Get)")) -> (s? t:f=w35:enum16{"Get", "Set", "Reset"})
      n244 = call "Status__LCR.vi"("Action (Get)"=w35, "Status In"=w37, "Bit"=u16 4) -> ("Status Out"=w39:u16)  [unwired: 7 in, 1 out]
      n245 = To Word Integer(number=w56) -> (16bit integer=w90:i16)
      n246 = Negate(x=w90) -> (-x=w30:i16)
      n247 = Bundle By Name(cluster=w49, "Status"=w39) -> (w23:T1)
      n248 = Select(t=w30, s=w25, f=i16 0) -> (s? t:f=w29:i16)
      n249 = call <vilib>:"InsetRect.vi"("dv"=w29, "dh"=w29, "rect"=w73) -> ("inset rect"=w72:T12)
      n250 = Unbundle By Name(w23) -> ("RunTimeSettings.Button Type"=w22:T6)
      n251 = Unbundle By Name(w72) -> ("left"=w71:i16, "top"=w70:i16)
      n252 = call <vilib>:"RectSize.vi"("rect"=w72) -> ("point"=w89:cluster{"x":i16, "y":i16})
      n253 = Bundle("left"=w71, "top"=w70) -> (w69:cluster{"left":i16, "top":i16})  [unwired: 1 in]
      n254 = case shown="\"Decoration\"" w22 {
        tunnel: w89 -> [w100 w110]
        tunnel: w88 -> [w94 w105]
        tunnel: [w99 w109] -> w83
        tunnel: [w98 w108] -> w81
        tunnel: w69 -> [w97 w107]
        tunnel: w51 -> [w95 w106]
        tunnel: w32 -> [w96 w101]
        frame Default {
          w91 = refnum<vi> refnum  # 布尔
          # "Set button size if shown"
          n255 = To More Specific Class(target class=w91, reference=w95, error in=w94) -> (specific class reference=w92:refnum<vi>, error out=w93:errorcluster)
          n256 = property class="Bool"(reference=w92, error in=w93, "Button Size"=w100, "Visible"=w96, "Position"=w97) -> (reference out=w98:refnum<vi>, error out=w99:errorcluster)
        }
        frame "Decoration" {
          w102 = refnum<vi> refnum  # 修饰
          # "Set button size if shown"
          n257 = To More Specific Class(target class=w102, reference=w106, error in=w105) -> (specific class reference=w103:refnum<vi>, error out=w104:errorcluster)
          n258 = property class="Decor"(reference=w103, error in=w104, "Size"=w110, "Visible"=w101, "Position"=w107) -> (reference out=w108:refnum<vi>, error out=w109:errorcluster)
        }
      }
      n259 = property class="GObj"(reference=w81, error in=w83) -> (reference out=w82:refnum<vi>, error out=w76:errorcluster, "Bounds"=w87:T11, "Position"=w84:T10)
      n260 = Compound Arithmetic op=ADD(w84, cluster{"Width":i32, "Height":i32} {"Width"=-3, "Height"=-3} ("Bounds")) -> (w67:T10)
      n261 = call "GetOwningPane__LCR.vi"("error in (no error)"=w76, "Control Reference"=w82) -> ("error out"=w79:errorcluster, "Owning Pane"=w80:refnum<vi>)  [unwired: 8 in]
      n262 = property on="Property Node" class="Pane"(reference=w80, error in=w79, "Origin"=w67) -> (error out=w78:errorcluster)  [unwired: 1 out]
      n263 = Add(x=w87, y=T11 {"Width"=6, "Height"=6} ("Bounds")) -> (x+y=w68:T11)
      n264 = property class="Ctl"(reference=w66, error in=w78, "Container Bounds"=w68) -> (error out=w77:errorcluster)  [unwired: 1 out]
      n265 = property class="Path"(reference=w65, "Position"=w67, "Size"=w68) -> ()  [unwired: 1 in, 2 out]
    }
    frame Error {
    }
  }
  "error out" <- w11
  "State Out" <- w6
  n266 = case shown="\"System\"" w1 {
    tunnel: "BX.FP Refs" -> [w534 w542 w550 w558]
    frame "Decoration" {
      n267 = Unbundle By Name(w534) -> ("SystemButton"=w533:refnum<vi>, "ModernButton"=w532:refnum<vi>, "ClassicButton"=w531:refnum<vi>)
      n268 = Build Array(w533, w532, w531) -> (w530:refnum<vi>[])
      n269 = for {
        tunnel: w530 -> [w536] mode=indexing
        n270 = property class="Bool"(reference=w536, "Visible"=FALSE) -> ()  [unwired: 1 in, 2 out]
      }
    }
    frame "Classic" {
      n271 = Unbundle By Name(w542) -> ("SystemButton"=w541:refnum<vi>, "ModernButton"=w540:refnum<vi>, "Decor Refnum"=w538:refnum<vi>)
      n272 = Build Array(w541, w540) -> (w539:refnum<vi>[])
      n273 = for {
        tunnel: w539 -> [w544] mode=indexing
        n274 = property class="Bool"(reference=w544, "Visible"=FALSE) -> ()  [unwired: 1 in, 2 out]
      }
      n275 = property class="Decor"(reference=w538, "Visible"=FALSE) -> ()  [unwired: 1 in, 2 out]
    }
    frame "Modern" {
      n276 = Unbundle By Name(w550) -> ("SystemButton"=w549:refnum<vi>, "ClassicButton"=w548:refnum<vi>, "Decor Refnum"=w546:refnum<vi>)
      n277 = Build Array(w549, w548) -> (w547:refnum<vi>[])
      n278 = for {
        tunnel: w547 -> [w552] mode=indexing
        n279 = property class="Bool (严格)"(reference=w552, "Visible"=FALSE) -> ()  [unwired: 1 in, 2 out]
      }
      n280 = property class="Decor"(reference=w546, "Visible"=FALSE) -> ()  [unwired: 1 in, 2 out]
    }
    frame "System" {
      n281 = Unbundle By Name(w558) -> ("ModernButton"=w557:refnum<vi>, "ClassicButton"=w556:refnum<vi>, "Decor Refnum"=w554:refnum<vi>)
      n282 = Build Array(w557, w556) -> (w555:refnum<vi>[])
      n283 = for {
        tunnel: w555 -> [w560] mode=indexing
        n284 = property class="Bool"(reference=w560, "Visible"=FALSE) -> ()  [unwired: 1 in, 2 out]
      }
      n285 = property class="Decor"(reference=w554, "Visible"=FALSE) -> ()  [unwired: 1 in, 2 out]
    }
  }
